vi "ReversedEngineering CountNoOfObjectAggregations.vi"(1 "Path":path, 4 "appended array":T1[](array[typedef]), 5 "error in (no error)":errorcluster) -> (15 "minAggregations":i32, 16 "anyFound":bool, 17 "noFoundLImit":bool, 19 "error out":errorcluster)   [LabVIEW 2012]
uses:
  <resource>/Framework/Providers/Open_GDS/UML/ReversedEngineering/ReversedEngineering AttributeInfoType.ctl
  <resource>/Framework/Providers/Open_GDS/UML/ReversedEngineering/ReversedEngineering AttributeDataType.ctl
  <resource>/Framework/Providers/Open_GDS/UML/UMLEditor/UMLEditor_VisibilityType.ctl
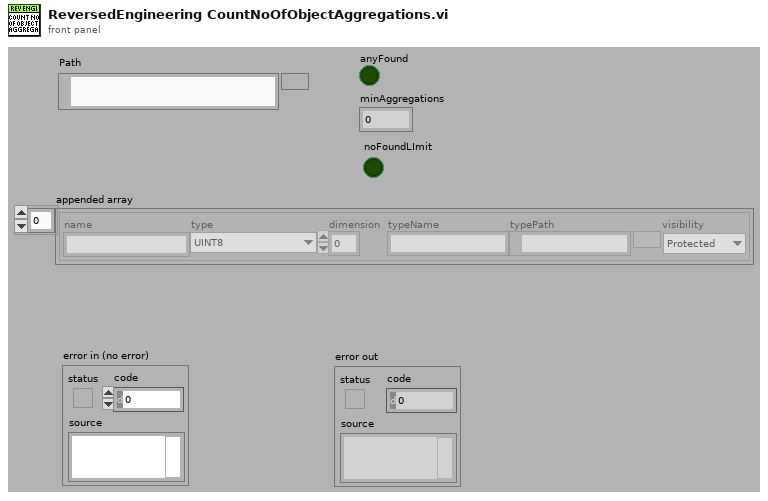
[diagram p1: front panel]
types:
  T1 = typedef "ReversedEngineering AttributeInfoType.ctl" = cluster{"name":string, "type":T2, "dimension":i32, "typeName":string, "typePath":path, "visibility":T3}
  T2 = typedef "ReversedEngineering AttributeDataType.ctl" = enum16{"UINT8", "INT8", "UINT16", "INT16", "UINT32", "INT32", "UINT64", "INT64", "SGL", "DBL", "EXT", "CSG", "CDB", "CXT", "TimeStamp", "STRING", "PATH", "BOOL", "ENUM", "RefNum", "VIRefNum", "ClassRefNum", "Cluster", "Variant", "TypeRef", "Waveform", "LabVIEW Object", "Other"}
  T3 = typedef "UMLEditor_VisibilityType.ctl" = enum16{"Public", "Private", "Protected"}
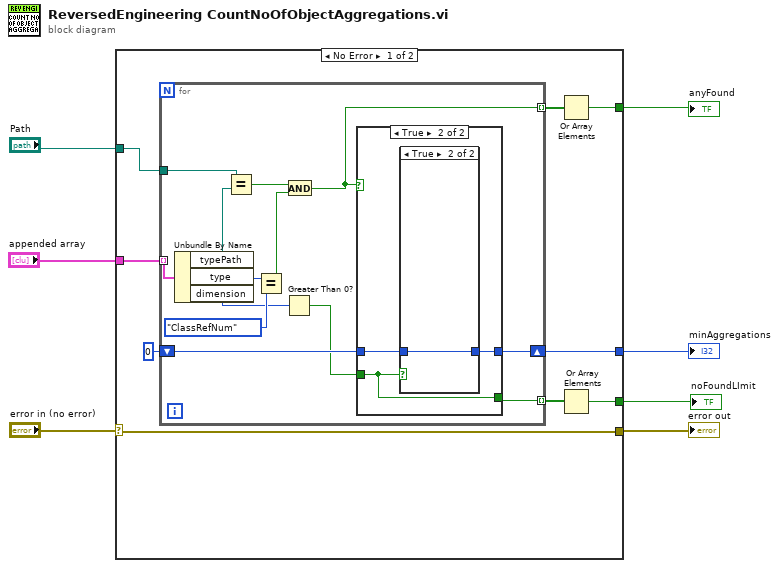
[diagram p0: block diagram]
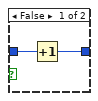
[diagram p3: hidden frame]
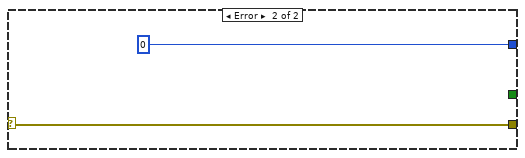
[diagram p4: hidden frame]
diagram:
  n1 = case shown="No Error" "error in (no error)" {
    selector: "error in (no error)" -> [w16 w38]
    tunnel: "Path" -> [w13 _]
    tunnel: [w16 w38] -> w6
    tunnel: [w14 u32 0] -> w4
    tunnel: [w11 _] -> w3
    tunnel: [w9 _] -> w2
    tunnel: "appended array" -> [w8 _]
    frame No Error {
      n2 = for {
        tunnel: w13 -> [w29]
        shift-right: [w28] -> w14
        shift-left: u32 0 -> [w25]
        tunnel: [w27] -> w12 mode=indexing
        tunnel: [w22] -> w10 mode=indexing
        tunnel: w8 -> [w26] mode=indexing
        n3 = Unbundle By Name(w26) -> ("typePath"=w24:path, "type"=w21:T2, "dimension"=w18:i32)
        n4 = Equal?(x=w29, y=w24) -> (x = y?=w23:bool)
        n5 = Equal?(x=w21, y=ReversedEngineering_AttributeDataType."ClassRefNum") -> (x = y?=w19:bool)
        n6 = Greater Than 0?(x=w18) -> (x > 0?=w17:bool)
        n7 = And(x=w23, y=w19) -> (x .and. y?=w22:bool)
        n8 = case shown="True" w22 {
          tunnel: w25 -> [w30 w33]
          tunnel: [w30 w32] -> w28
          tunnel: w17 -> [_ w31]
          tunnel: [_ w31] -> w27
          frame False {
          }
          frame True {
            n9 = case shown="True" w31 {
              tunnel: w33 -> [w35 w36]
              tunnel: [w34 w36] -> w32
              frame False {
                n10 = Increment(x=w35) -> (x+1=w34:u32)
              }
              frame True {
              }
            }
          }
        }
      }
      n11 = Or Array Elements(Boolean array=w10) -> (logical OR=w9:bool)
      n12 = Or Array Elements(Boolean array=w12) -> (logical OR=w11:bool)
    }
    frame Error {
    }
  }
  "error out" <- w6
  "minAggregations" <- w4
  "anyFound" <- w2
  "noFoundLImit" <- w3
